vi "BGSub.vi"(8 "error in (no error)":errorcluster, 10 "BG IN":T1, 11 "raw Image In":T1) -> (0 "error out":errorcluster, 3 "Refnum out":T1, 4 "empty image":bool)   [LabVIEW 2011]
uses:
  IMAQ Image.ctl
  NI_Vision_Development_Module.lvlib
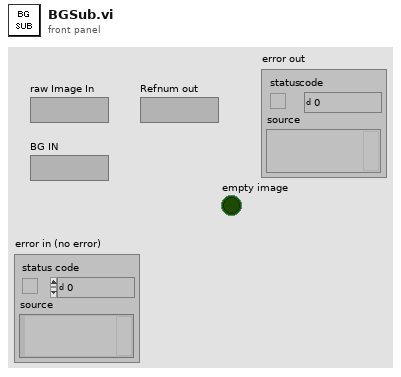
[diagram p1: front panel]
types:
  T1 = typedef "IMAQ Image.ctl" = refnum<image>
  T2 = typedef "Image Type" = u32
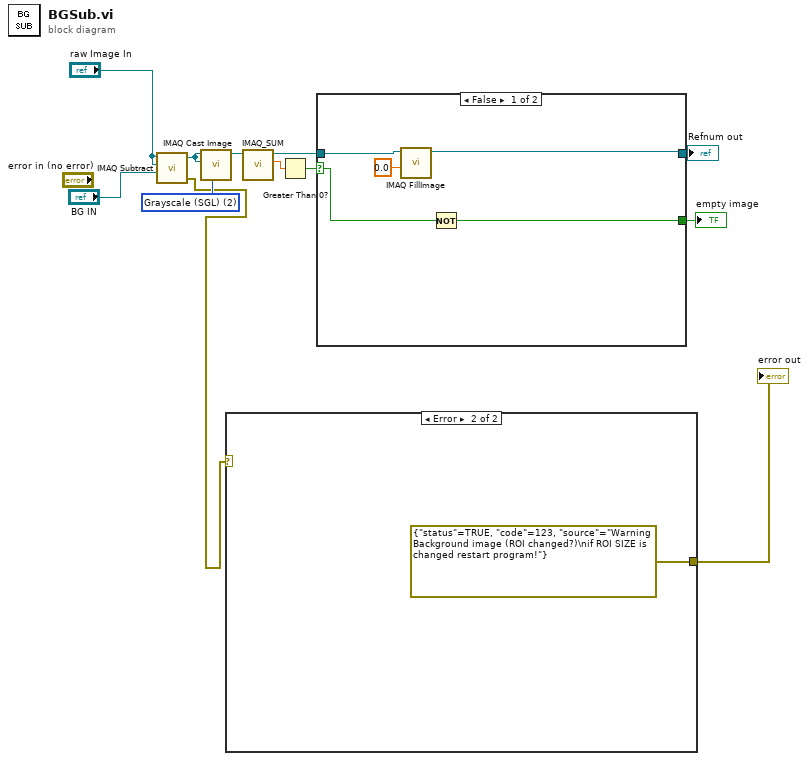
[diagram p0: block diagram]
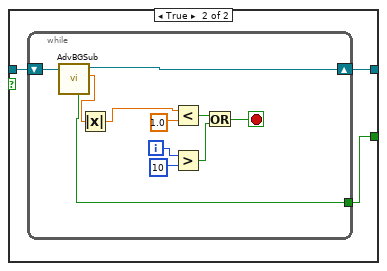
[diagram p3: hidden frame]
diagram:
  w8 = T2 2 items=["Grayscale (U8)", "Grayscale (I16)", "Grayscale (SGL)", "Complex (CSG)", "RGB (U32)", "HSL (U32)", "RGB (U64)", "Grayscale (U16)"] ("Image Type")
  n1 = call "IMAQ Subtract"("Image Src A"="raw Image In", "Image Dst"="raw Image In", "Image Src B"="BG IN") -> ("Image Dst Out"=w7:T1, "error out"=w3:errorcluster)  [unwired: 4 in]
  n2 = call "IMAQ Cast Image"("Image Type"=w8, "Image Dst"=w7, "Image Src"=w7) -> ("Image Dst Out"=w9:T1)  [unwired: 7 in, 1 out]
  n3 = case shown="Error" w3 {
    selector: w3 -> [w13 _]
    tunnel: [w13 errorcluster {"status"=TRUE, "code"=123, "source"="Warning Background image (ROI changed?)\nif ROI SIZE is changed restart program!"} ("error out")] -> w2
    frame No Error {
    }
    frame Error {
    }
  }
  "error out" <- w2
  n4 = call "IMAQ_SUM.vi"("Image"=w9) -> ("Sum"=w10:sgl, "Image 2"=w11:T1)  [unwired: 9 in]
  n5 = Greater Than 0?(x=w10) -> (x > 0?=w12:bool)
  n6 = case shown="False" w12 {
    selector: w12 -> [w16 _]
    tunnel: [w17 w22] -> w6
    tunnel: w11 -> [w19 w21]
    tunnel: [w15 w20] -> w1
    frame False {
      n7 = call "IMAQ FillImage"("Pixel Value (U8, U16, I16, Float)"=sgl 0.0, "Image"=w19) -> ("Image Out"=w17:T1)  [unwired: 8 in, 1 out]
      n8 = Not(x=w16) -> (.not. x?=w15:bool)
    }
    frame True {
      n9 = while {
        shift-right: [w33] -> w22
        shift-left: w21 -> [w32]
        tunnel: [w23] -> w20
        i -> [w31]
        stop <- w30 stop-if-true
        n10 = call "AdvBGSub.vi"("Refnum in"=w32) -> ("-x"=w25:sgl, "Refnum out"=w33:T1, "empty image"=w23:bool)  [unwired: 7 in, 1 out]
        n11 = Absolute Value(x=w25) -> (abs(x)=w24:sgl)
        n12 = Less?(x=w24, y=sgl 1.0) -> (x < y?=w28:bool)
        n13 = Greater?(x=w31, y=10) -> (0:w26:bool)
        n14 = Or(x=w28, y=w26) -> (x .or. y?=w30:bool)
      }
    }
  }
  "Refnum out" <- w6
  "empty image" <- w1
